vi "Transcriptor LabVIEW to Python code Step 3 Translate Elements.vi"(8 "error in (no error)":errorcluster, 10 "reentrant VIs":string[](array[string]), 11 "Diagram in":refnum<vi>) -> (0 "error out":errorcluster, 1 "transcripted C code":string[](array[string]), 2 "feedback assignments":string[](array[string]), 3 "transcriptor cluster":T1[](array[typedef]))   [LabVIEW 2018]
uses:
  types/LabVIEW Universal Transcriptor Cluster.ctl
  <vilib>/Utility/miscctls.llb/LVPointTypeDef.ctl
  <vilib>/regexp/Match Regular Expression.xnode
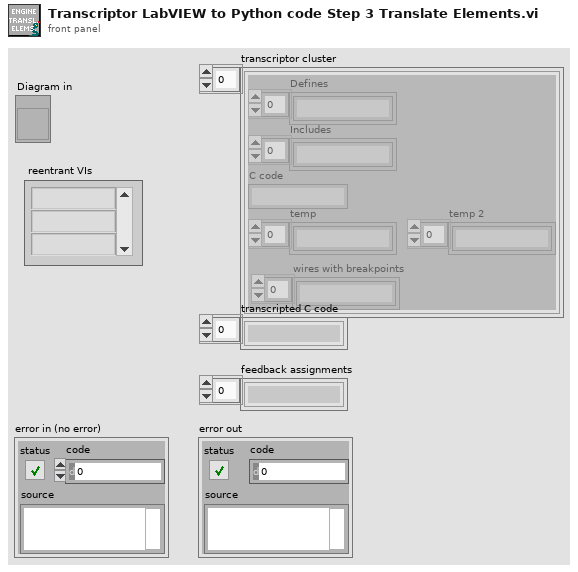
[diagram p1: front panel]
types:
  T1 = typedef "LabVIEW Universal Transcriptor Cluster.ctl" = cluster{"Defines":string[], "Includes":string[], "C code":string, "temp":string[], "temp 2":string[], "wires with breakpoints":string[]}
  T2 = typedef "LVPointTypeDef.ctl" = cluster{"Horizontal":i16, "Vertical":i16}
  T3 = cluster{"wire labels":string[], "wire terminals datatypes":string[][]}
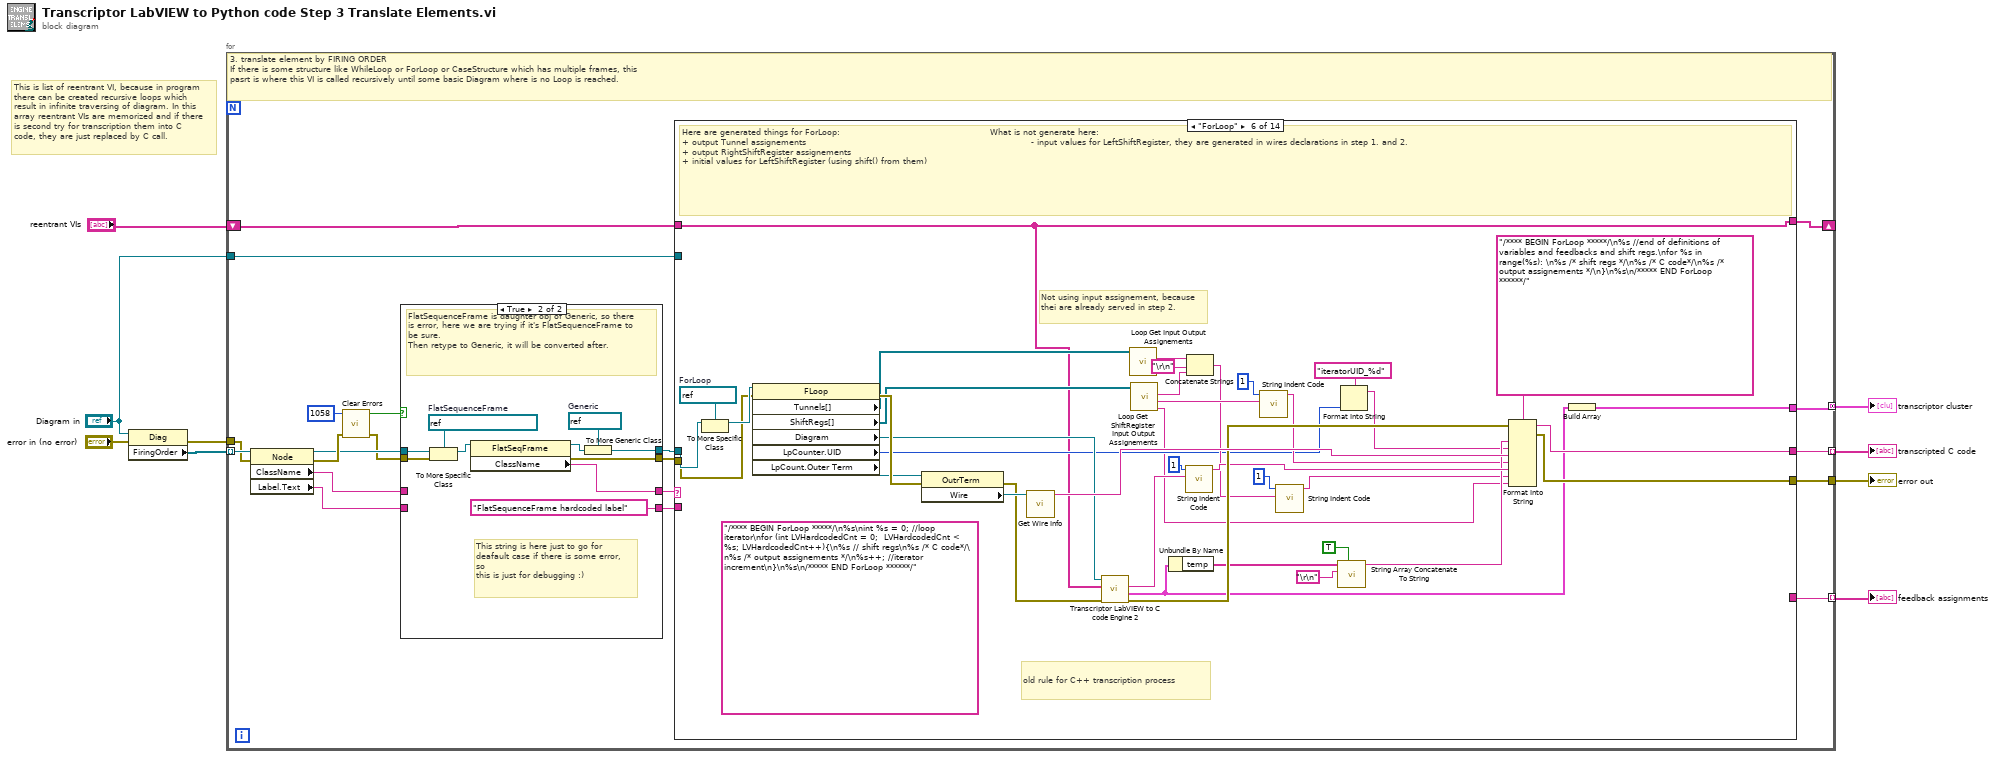
[diagram p0: block diagram]
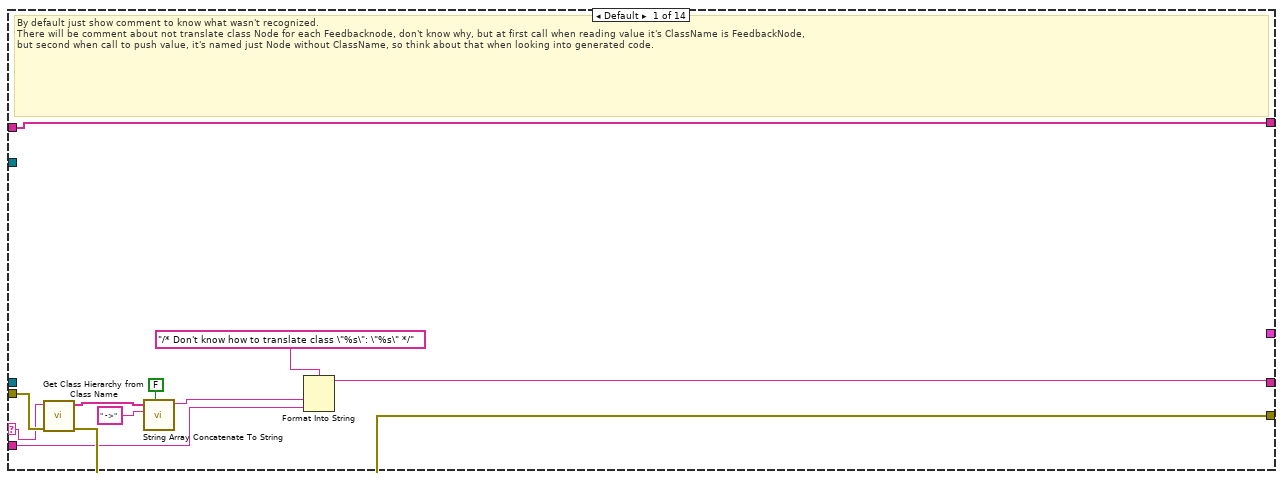
[diagram p3: hidden frame]
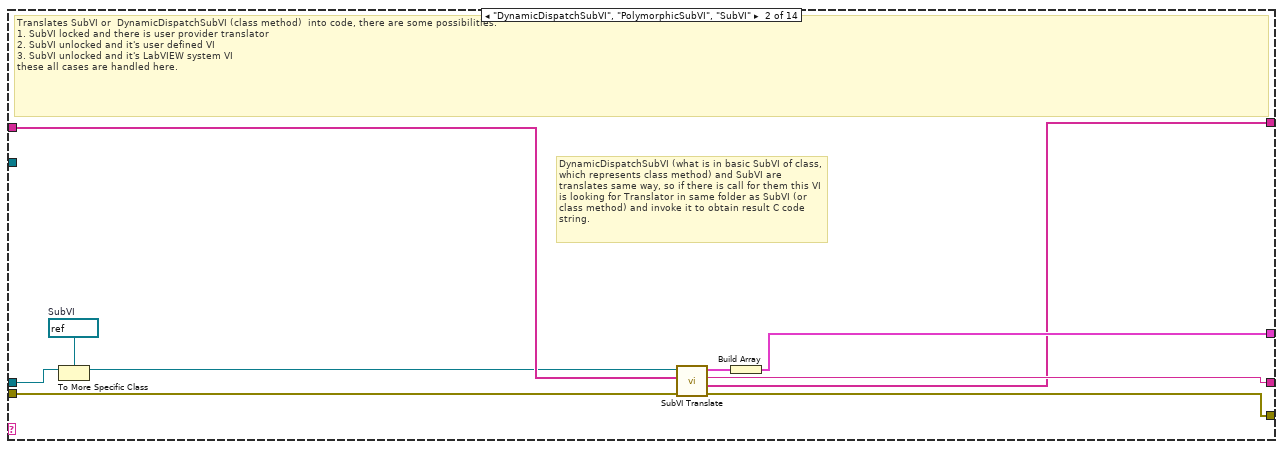
[diagram p4: hidden frame]
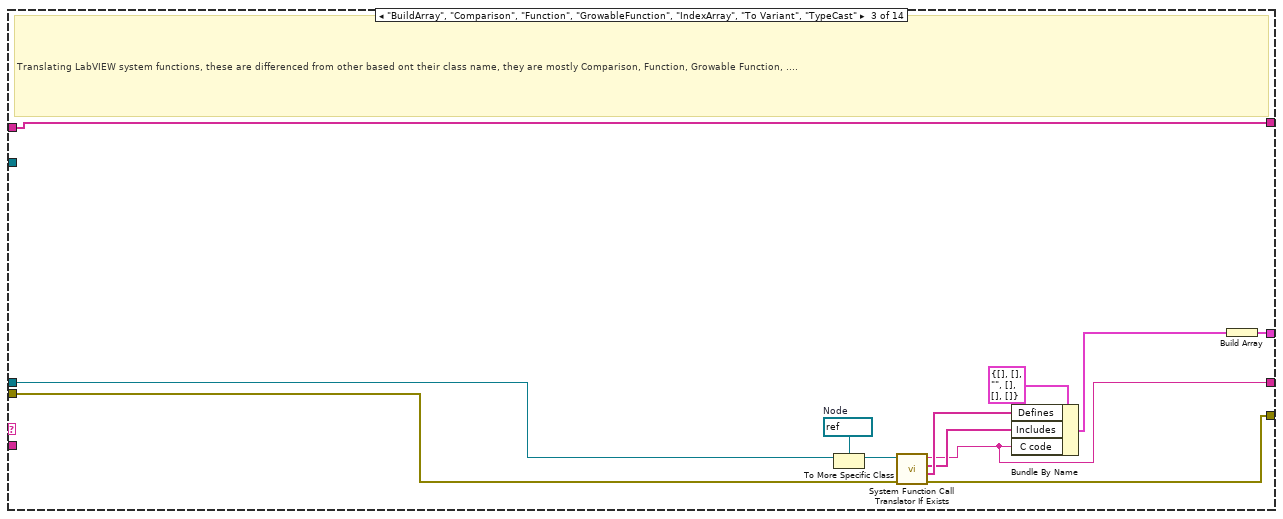
[diagram p5: hidden frame]
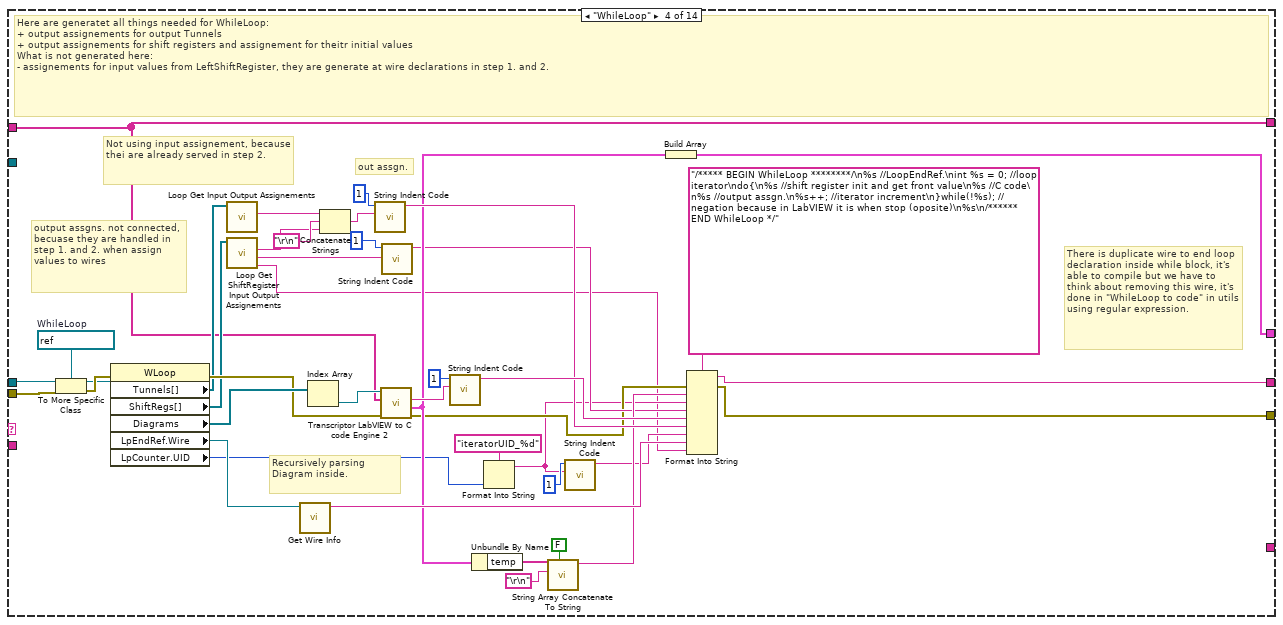
[diagram p6: hidden frame]
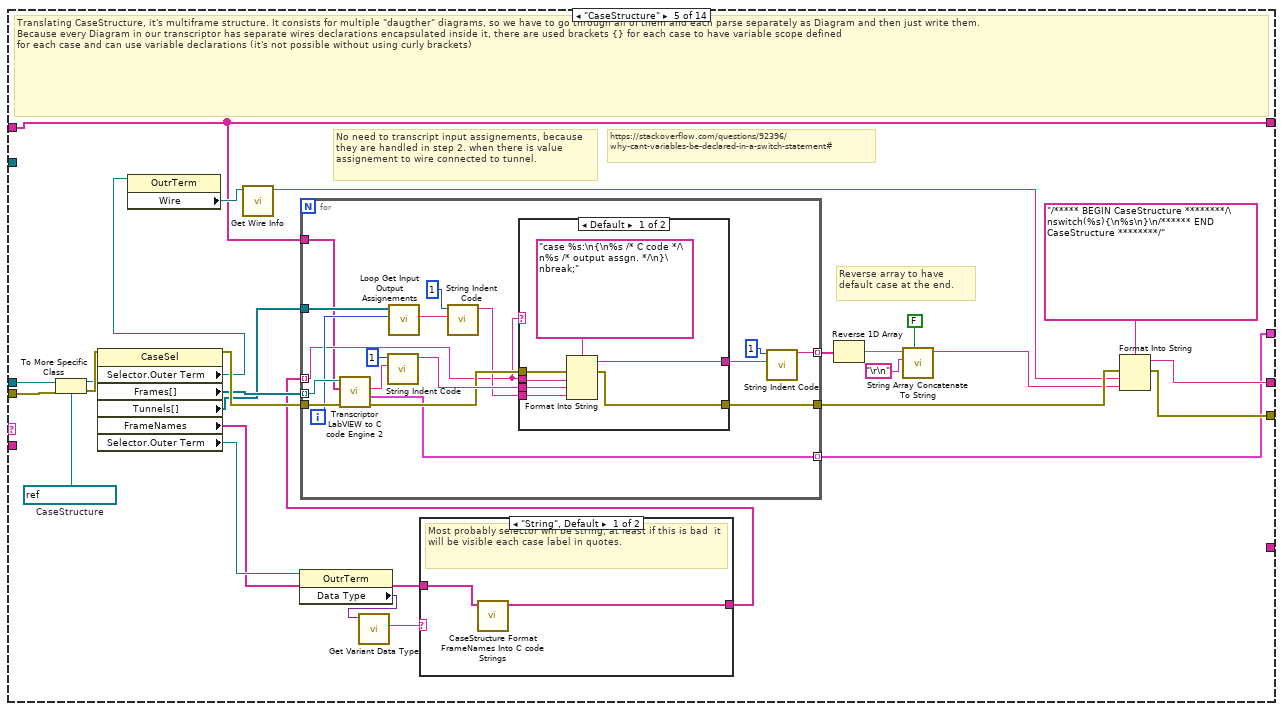
[diagram p7: hidden frame]
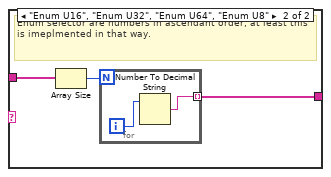
[diagram p8: hidden frame]
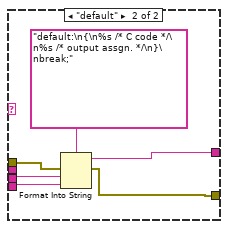
[diagram p9: hidden frame]
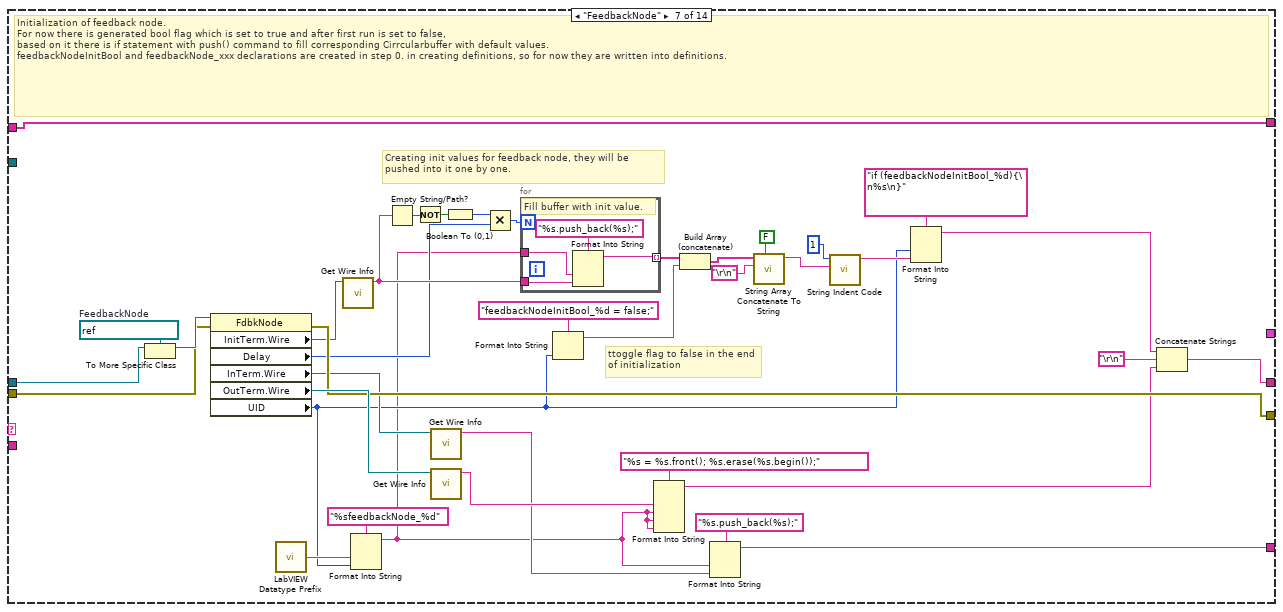
[diagram p10: hidden frame]
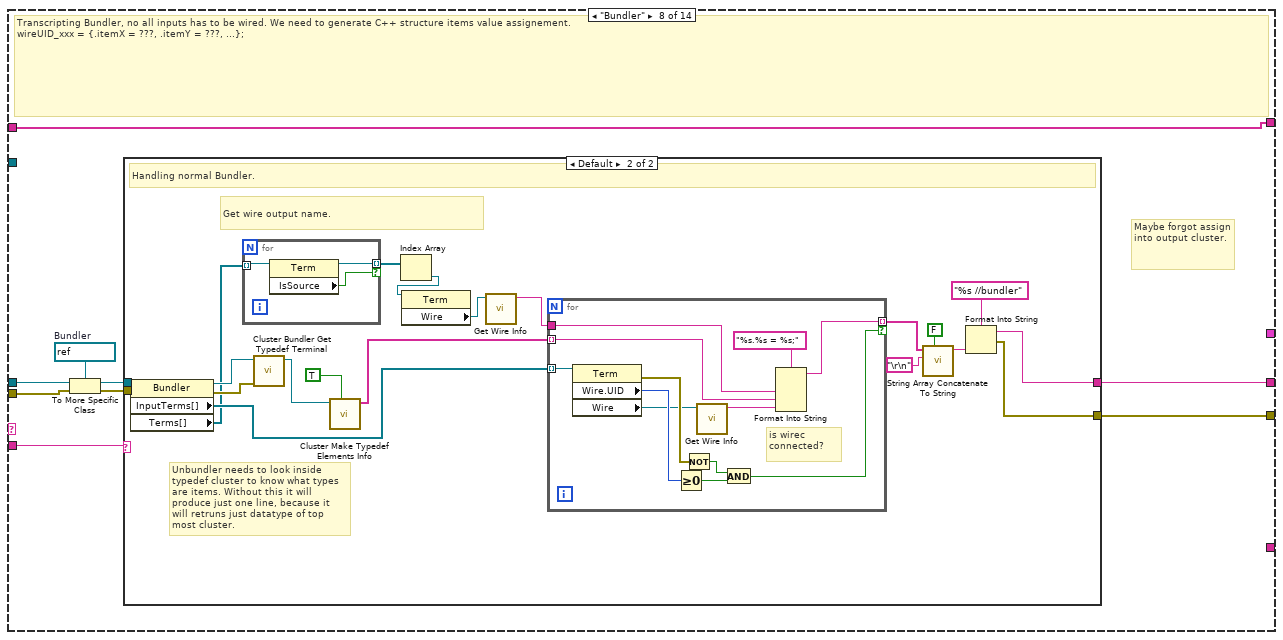
[diagram p11: hidden frame]
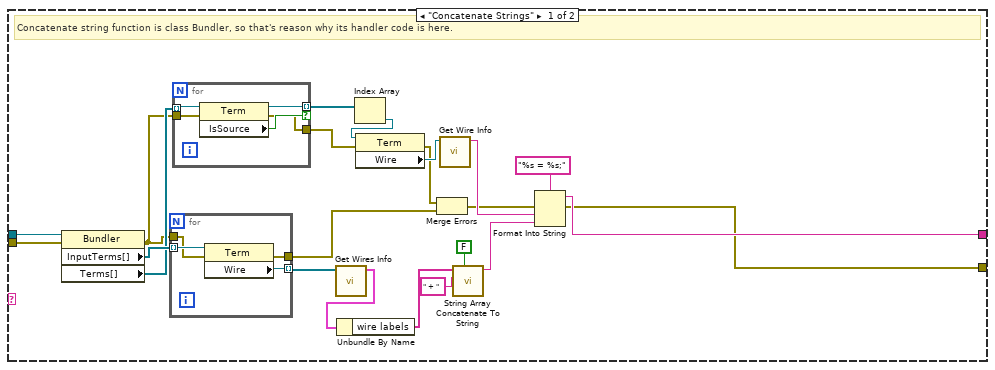
[diagram p12: hidden frame]
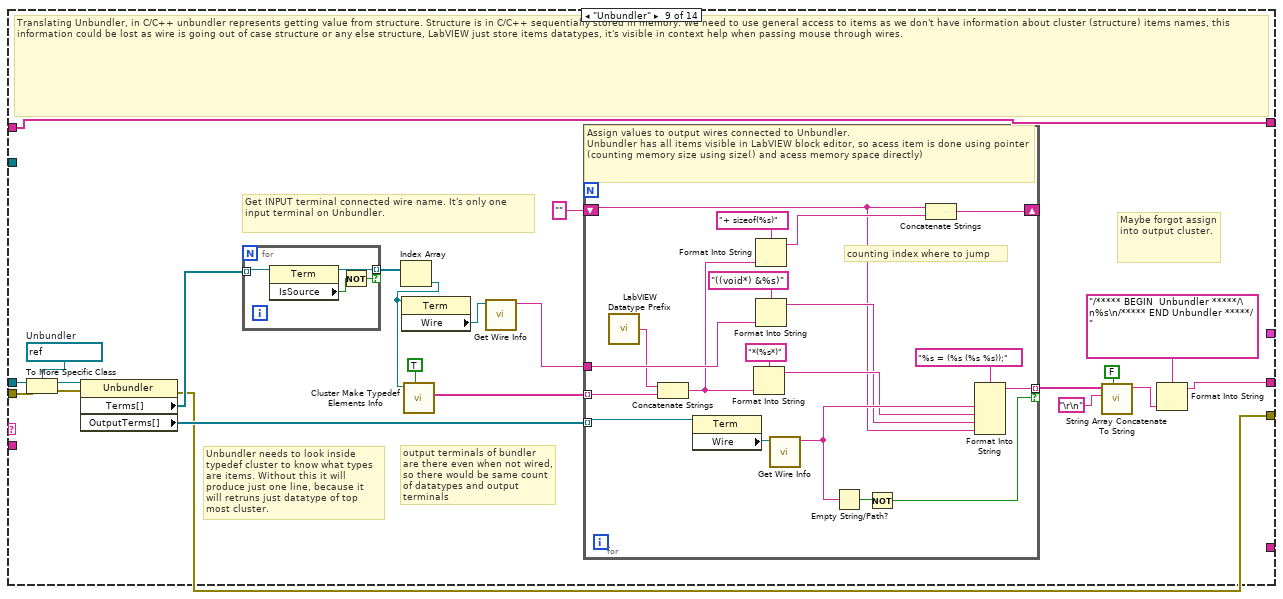
[diagram p13: hidden frame]
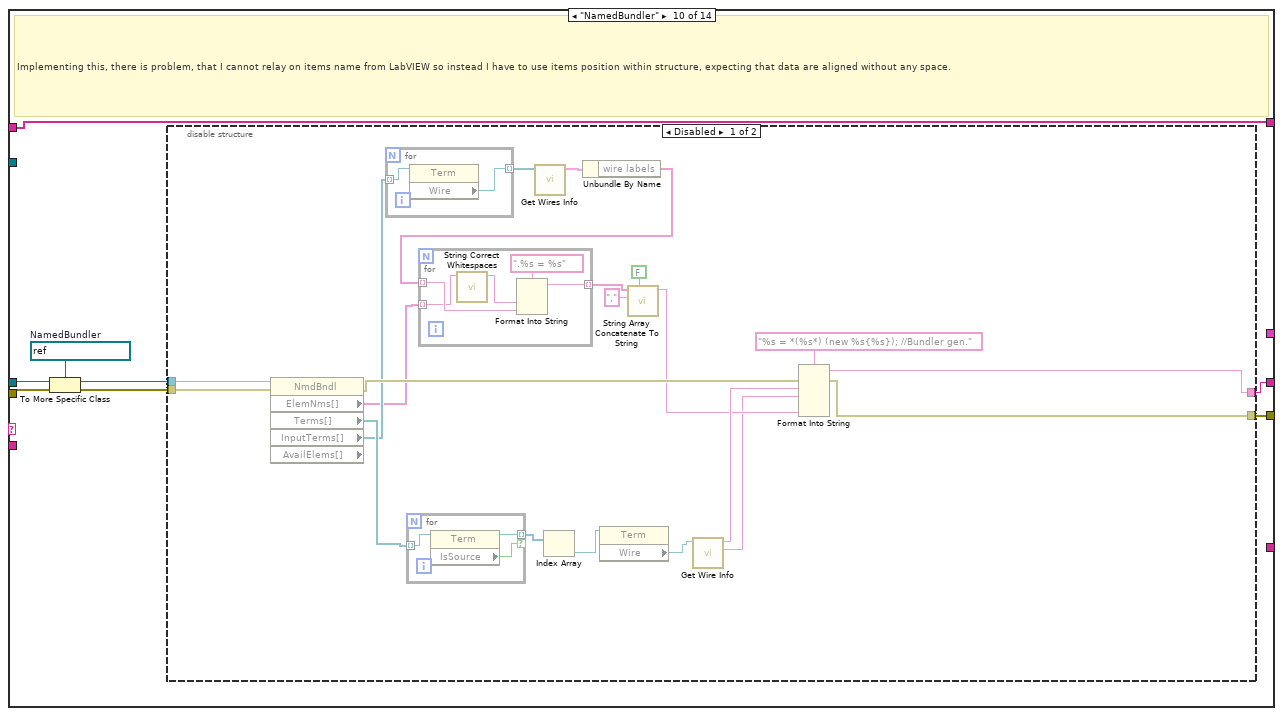
[diagram p14: hidden frame]
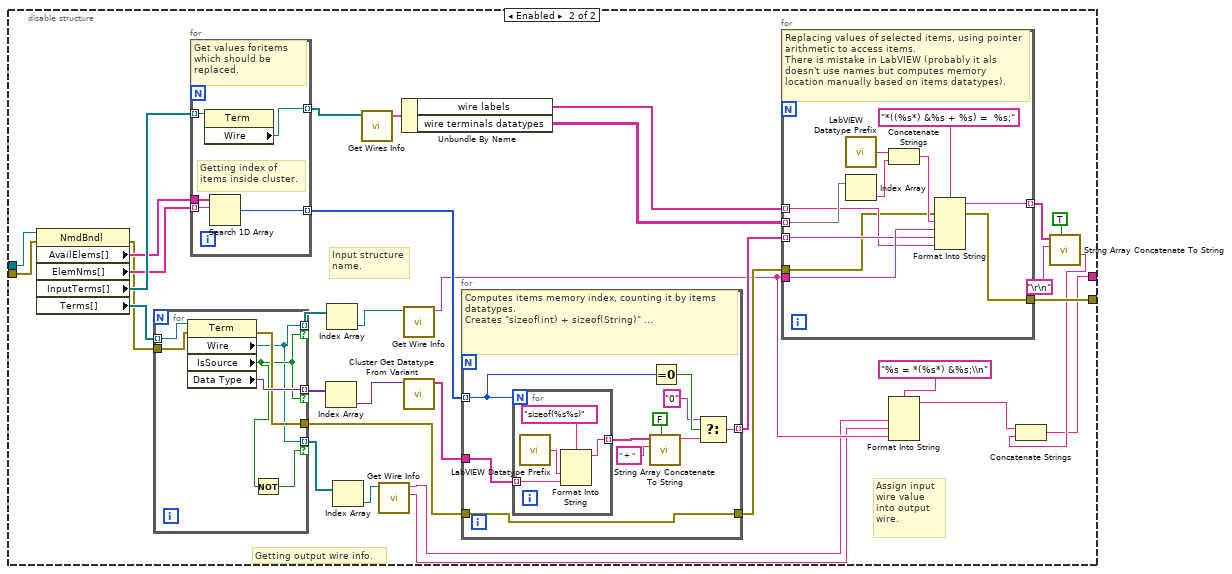
[diagram p15: hidden frame]
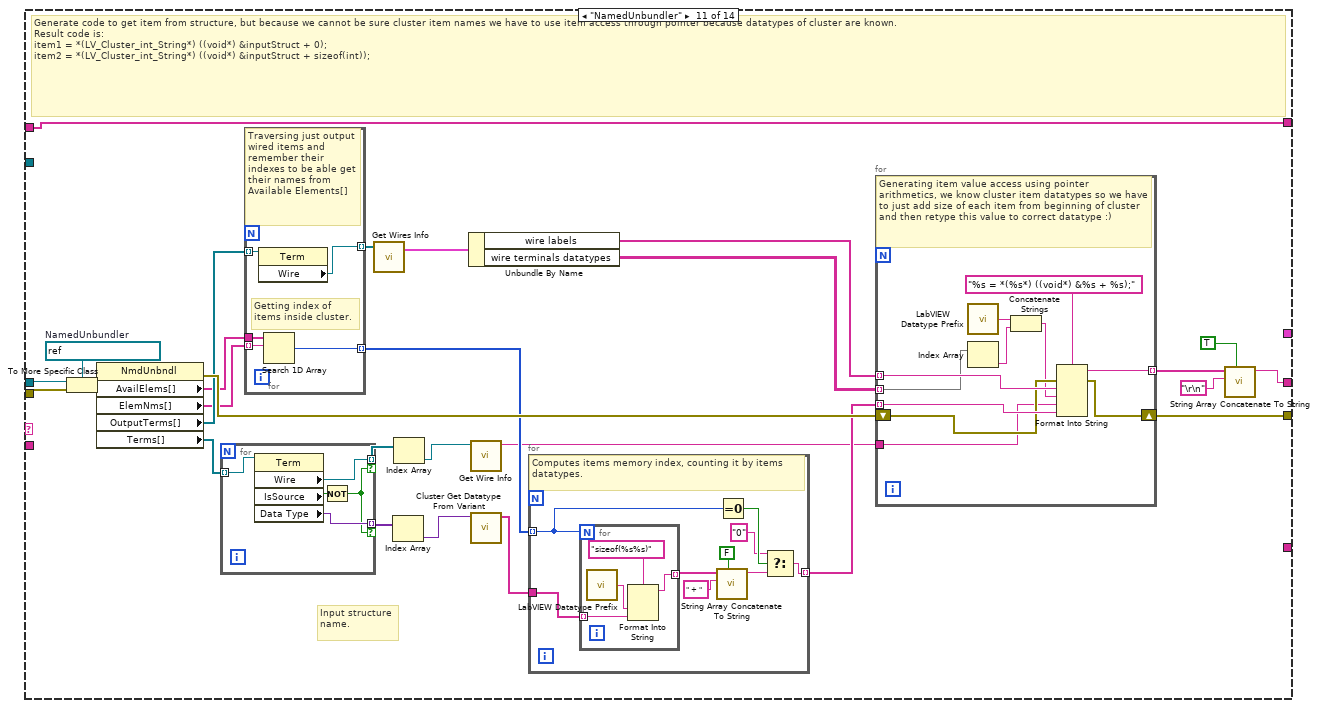
[diagram p16: hidden frame]
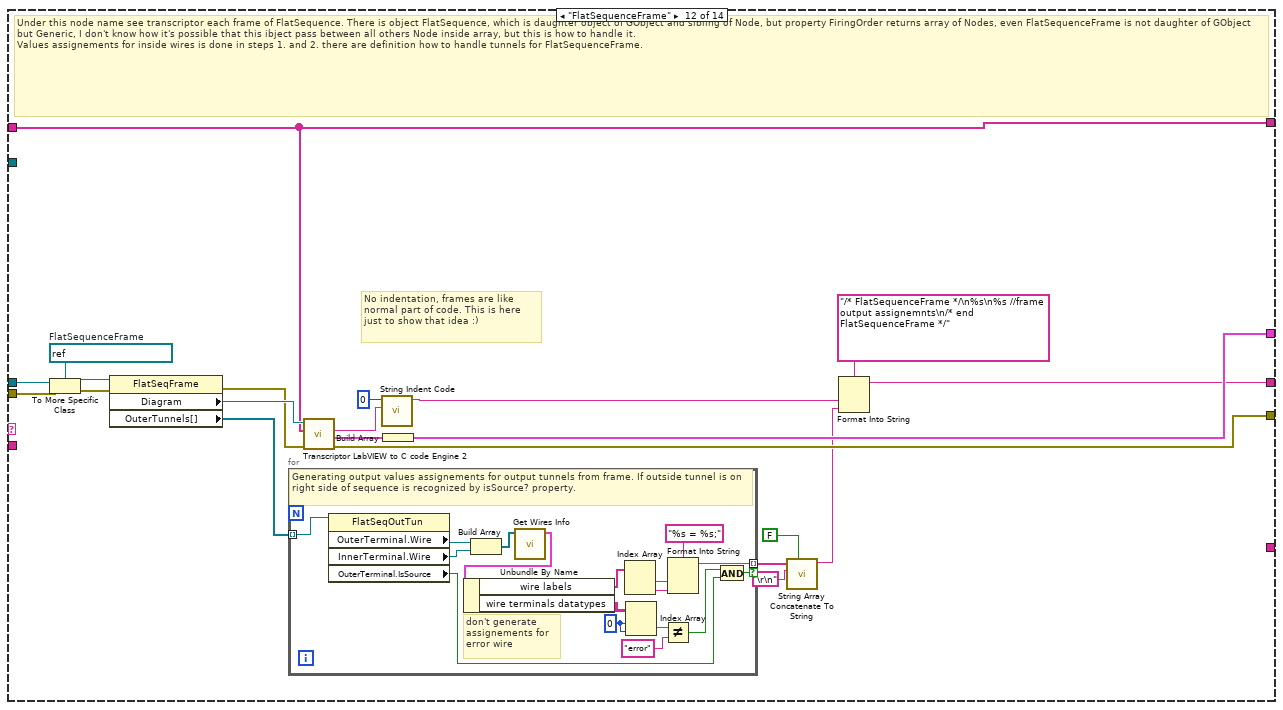
[diagram p17: hidden frame]
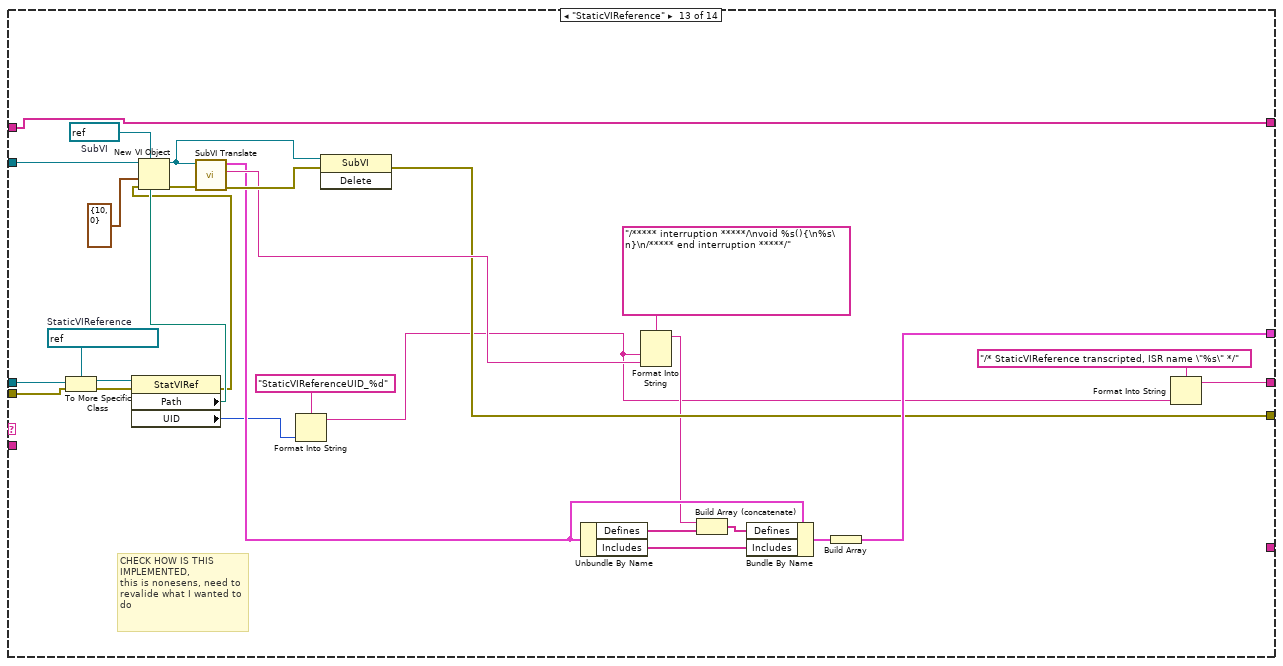
[diagram p18: hidden frame]
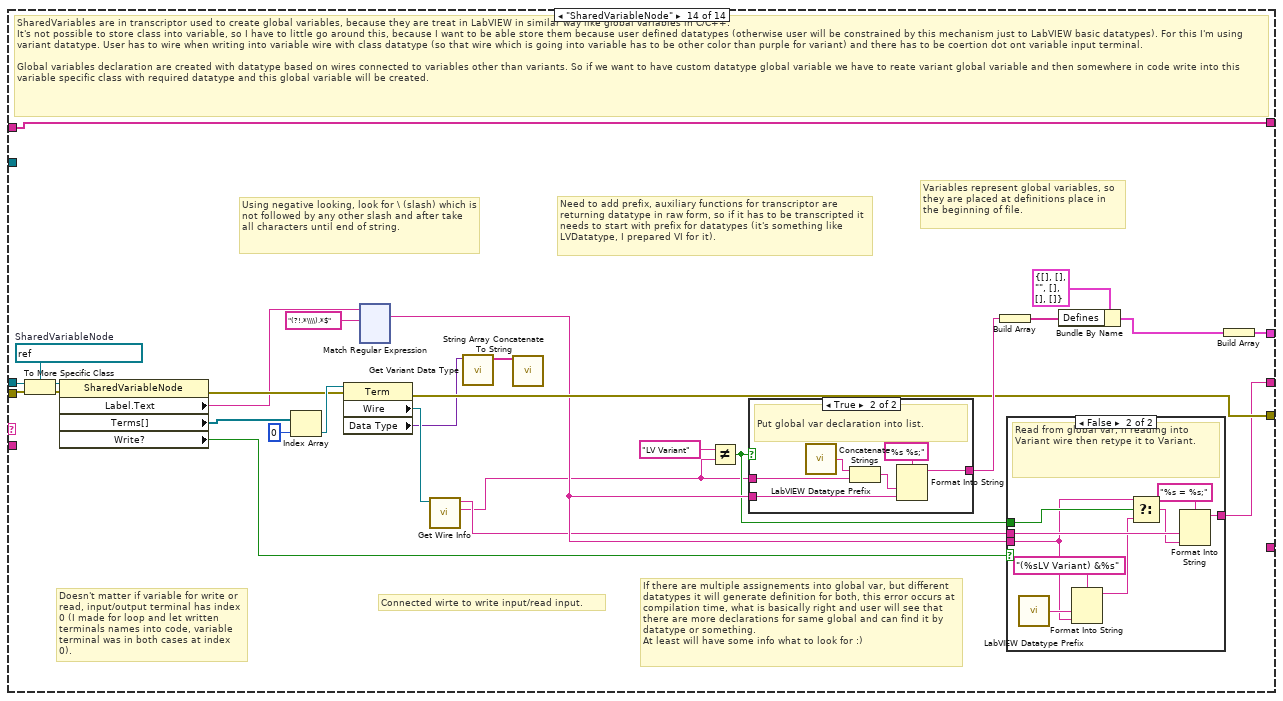
[diagram p19: hidden frame]
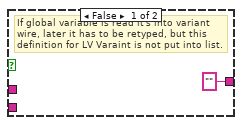
[diagram p20: hidden frame]
diagram:
  # "This is list of reentrant VI, because in program there can be created recursive loops which result in infinite traversing of diagram. In this array reentrant VIs are memorized and if there is second try for transcription them into C code, they are just replaced by C call."
  n1 = property on="Property Node" class="Diag"(reference="Diagram in", error in="error in (no error)") -> (error out=w4:errorcluster, "FiringOrder"=w9:refnum<vi>[])  [unwired: 1 out]
  n2 = for {
    tunnel: w9 -> [w29] mode=indexing
    tunnel: w4 -> [w28]
    tunnel: [w25] -> w5 mode=indexing
    tunnel: [w24] -> w7
    tunnel: [w27] -> w3 mode=concatenating
    tunnel: [w26] -> w8 mode=indexing
    tunnel: "Diagram in" -> [w12]
    shift-right: [w11] -> _
    shift-left: "reentrant VIs" -> [w10]
    # "3. translate element by FIRING ORDER\nIf there is some structure like WhileLoop or ForLoop or CaseStructure which has multiple frames, this\npasrt is where this VI is called recursively until some basic Diagram where is no Loop is reached."
    n3 = property class="Node"(reference=w29, error in=w28) -> (reference out=w21:refnum<vi>, error out=w23:errorcluster, "ClassName"=w16:string, "Label.Text"=w15:string)
    n4 = call <vilib>:"Clear Errors.vi"("error in (no error)"=w23, "specific error code to clear (0: all)"=1058) -> ("error out"=w20:errorcluster, "specific error cleared?"=w19:bool)  [unwired: 4 in]
    n5 = case shown="True" w19 {
      tunnel: w21 -> [w30 w43]
      tunnel: w20 -> [w31 w42]
      tunnel: [w33 w39] -> w18
      tunnel: [w32 "FlatSequenceFrame hardcoded label" ("Label.Text")] -> w17
      tunnel: w16 -> [w33 _]
      tunnel: w15 -> [w32 _]
      tunnel: [w31 w38] -> w14
      tunnel: [w30 w34] -> w13
      frame False {
        # "No error, so we are parsing some Node."
      }
      frame True {
        w36 = refnum<vi> refnum  # Generic
        w41 = refnum<vi> refnum  # FlatSequenceFrame
        # "This string is here just to go for\ndeafault case if there is some error, so\nthis is just for debugging :)"
        # "FlatSequenceFrame is daughter obj of Generic, so there is error, here we are trying if it's FlatSequenceFrame to be sure.\nThen retype to Generic, it will be converted after."
        n6 = To More Specific Class(target class=w41, reference=w43, error in=w42) -> (specific class reference=w40:refnum<vi>)  [unwired: 1 out]
        n7 = property class="FlatSeqFrame"(reference=w40) -> (reference out=w35:refnum<vi>, error out=w38:errorcluster, "ClassName"=w39:string)  [unwired: 1 in]
        n8 = To More Generic Class(target class=w36, reference=w35) -> (generic class reference=w34:refnum<vi>)
      }
    }
    n9 = case shown="\"ForLoop\"" w18 {
      selector: w18 -> [w45 _ _ _ _ _ _ _ _ _ _ _ _ _]
      tunnel: w13 -> [_ w57 w68 w117 w127 w221 w259 w271 w357 w391 w520 w575 w620 w648]
      tunnel: [w53 w64 w73 w109 w139 w211 w232 w266 w341 w385 w506 w561 w597 w626] -> w25
      tunnel: w14 -> [w48 w60 w76 w113 w142 w218 w251 w270 w356 w390 w519 w571 w619 w649]
      tunnel: [w47 w63 w70 w108 w137 w212 w250 w267 w344 w386 w514 w565 w605 w636] -> w24
      tunnel: [_ w61 w72 w98 w126 w203 _ _ _ _ _ w563 w616 w642] -> w27
      tunnel: w17 -> [w46 _ _ _ _ _ _ w265 _ _ _ _ _ _]
      tunnel: [_ _ _ _ _ _ w226 _ _ _ _ _ _ _] -> w26
      tunnel: w12 -> [_ _ _ _ _ _ _ _ _ _ _ _ w614 _]
      tunnel: w10 -> [w44 w59 w65 w78 w123 w184 w222 w264 w340 w384 w493 w555 w593 w644]
      tunnel: [w44 w58 w65 w78 w123 w184 w222 w264 w340 w384 w493 w555 w593 w644] -> w11
      frame Default {
        # "By default just show comment to know what wasn't recognized.\nThere will be comment about not translate class Node for each Feedbacknode, don't know why, but at first call when reading value it's ClassName is FeedbackNode,\nbut second when call to push value, it's named just Node without ClassName, so think about that when looking into generated code."
        n10 = call <vilib>:"Get Class Hierarchy from Class Name.vi"("error in (no error)"=w48, "Class Name"=w45) -> ("error out"=w47:errorcluster, "Class Hierarchy"=w51:string[])  [unwired: 8 in]
        n11 = call "String Array Concatenate To String.vi"("insert last delimiter?"=FALSE, "Delimiter char"=" ->", "Array String In"=w51) -> ("String"=w49:string)  [unwired: 8 in]
        n12 = Format Into String(format string="/* Don't know how to translate class \"%s\": \"%s\" */", w49, w46) -> (resulting string=w53:string)  [unwired: 2 in, 1 out]
      }
      frame "DynamicDispatchSubVI", "PolymorphicSubVI", "SubVI" {
        w55 = refnum<vi> refnum  # SubVI
        # "DynamicDispatchSubVI (what is in basic SubVI of class, which represents class method) and SubVI are translates same way, so if there is call for them this VI is looking for Translator in same folder as SubVI (or class method) and invoke it to obtain result C code string."
        # "Translates SubVI or  DynamicDispatchSubVI (class method)  into code, there are some possibilities:\n1. SubVI locked and there is user provider translator\n2. SubVI unlocked and it's user defined VI\n3. SubVI unlocked and it's LabVIEW system VI\nthese all cases are handled here."
        n13 = To More Specific Class(target class=w55, reference=w57) -> (specific class reference=w56:refnum<vi>)  [unwired: 1 in, 1 out]
        n14 = call "SubVI Translate.vi"("error in (no error)"=w60, "reentrant VIs"=w59, "SubVI in"=w56) -> ("error out"=w63:errorcluster, "reentrant VIs out"=w58:string[], "transcripted code"=w64:string, "transcriptor cluster"=w62:T1)  [unwired: 5 in]
        n15 = Build Array(w62) -> (w61:T1[])
      }
      frame "BuildArray", "Comparison", "Function", "GrowableFunction", "IndexArray", "To Variant", "TypeCast" {
        w66 = refnum<vi> refnum  # Node
        # "Translating LabVIEW system functions, these are differenced from other based ont their class name, they are mostly Comparison, Function, Growable Function, ...."
        n16 = To More Specific Class(target class=w66, reference=w68) -> (specific class reference=w67:refnum<vi>)  [unwired: 1 in, 1 out]
        n17 = call "System Function Call Translator If Exists.vi"("Error In"=w76, "Node Refnum"=w67) -> ("Error Out"=w70:errorcluster, "Defines"=w75:string[], "Includes"=w74:string[], "Replaced Code"=w73:string)  [unwired: 6 in]
        n18 = Bundle By Name(cluster=T1 {"Defines"=[], "Includes"=[], "C code"="", "temp"=[], "temp 2"=[], "wires with breakpoints"=[]} ("input cluster"), "Defines"=w75, "Includes"=w74, "C code"=w73) -> (w71:T1)
        n19 = Build Array(w71) -> (w72:T1[])
      }
      frame "WhileLoop" {
        w116 = refnum<vi> refnum  # WhileLoop
        # "output assgns. not connected, becuase they are handled in step 1. and 2. when assign values to wires"
        # "Not using input assignement, because thei are already served in step 2."
        # "out assgn."
        # "There is duplicate wire to end loop declaration inside while block, it's able to compile but we have to think about removing this wire, it's done in \"WhileLoop to code\" in utils using regular expression."
        # "Recursively parsing Diagram inside."
        # "Here are generatet all things needed for WhileLoop:\n+ output assignements for output Tunnels\n+ output assignements for shift registers and assignement for theitr initial values\nWhat is not generated here:\n- assignements for input values from LeftShiftRegister, they are generate at wire declarations in step 1. and 2."
        n20 = To More Specific Class(target class=w116, reference=w117, error in=w113) -> (specific class reference=w107:refnum<vi>, error out=w115:errorcluster)
        n21 = property class="WLoop"(reference=w107, error in=w115) -> (error out=w112:errorcluster, "Tunnels[]"=w102:refnum<vi>[], "ShiftRegs[]"=w89:refnum<vi>[], "Diagrams"=w114:refnum<vi>[], "LpEndRef.Wire"=w106:refnum<vi>, "LpCounter.UID"=w82:i32)  [unwired: 1 out]
        n22 = call "Loop Get Input Output Assignements.vi"("Loop Tunnels[]"=w102) -> ("tunnels output assignements"=w93:string)  [unwired: 9 in, 1 out]
        n23 = call "Loop Get ShiftRegister Input Output Assignements.vi"("RightShiftRegister[]"=w89) -> ("right shift regs outside wires assgn."=w77:string, "init values"=w79:string, "output assignements"=w88:string)  [unwired: 7 in, 1 out]
        n24 = call "Get Wire Info.vi"("Wire"=w106) -> ("wire label"=w101:string)  [unwired: 9 in, 1 out]
        n25 = Index Array(array=w114) -> (element=w111:refnum<vi>)  [unwired: 1 in]
        n26 = Concatenate Strings(w93, "\r\n", w88) -> (w91:string)
        n27 = call "String Indent Code.vi"("complete code"=w91, "actual nested level"=1) -> ("indented code"=w99:string)  [unwired: 9 in]
        n28 = call "Transcriptor LabVIEW to C code Engine 2.vi"("Error In"=w112, "List Reentrant VIs"=w78, "Diagram in"=w111) -> ("error out"=w85:errorcluster, "output cluster"=w97:T1, "transcripted code"=w105:string)  [unwired: 4 in, 2 out]
        n29 = call "String Indent Code.vi"("complete code"=w79, "actual nested level"=1) -> ("indented code"=w86:string)  [unwired: 9 in]
        n30 = call "String Indent Code.vi"("complete code"=w105, "actual nested level"=1) -> ("indented code"=w103:string)  [unwired: 9 in]
        n31 = Unbundle By Name(w97) -> ("temp"=w96:string[])
        n32 = Format Into String(format string="iteratorUID_%d", w82) -> (resulting string=w80:string)  [unwired: 2 in, 1 out]
        n33 = call "String Array Concatenate To String.vi"("insert last delimiter?"=FALSE, "Delimiter char"="\r\n", "Array String In"=w96) -> ("String"=w90:string)  [unwired: 8 in]
        n34 = call "String Indent Code.vi"("complete code"=w80, "actual nested level"=1) -> ("indented code"=w81:string)  [unwired: 9 in]
        n35 = Build Array(w97) -> (w98:T1[])
        n36 = Format Into String(format string="/***** BEGIN WhileLoop ********/\n%s //LoopEndRef.\nint %s = 0; //loop iterator\ndo{\n%s //shift register init and get front value\n%s //C code\n%s //output assgn.\n%s++; //iterator increment\n}while(!%s); //negation because in LabVIEW it is when stop (oposite)\n%s\n/****** END WhileLoop */", error in=w85, w90, w80, w86, w103, w99, w81, w101, w77) -> (resulting string=w109:string, error out=w108:errorcluster)  [unwired: 1 in]
      }
      frame "CaseStructure" {
        w144 = refnum<vi> refnum  # CaseStructure
        # "Reverse array to have default case at the end."
        # "https://stackoverflow.com/questions/92396/why-cant-variables-be-declared-in-a-switch-statement#"
        # "No need to transcript input assignements, because they are handled in step 2. when there is value assignement to wire connected to tunnel."
        # "Translating CaseStructure, it's multiframe structure. It consists for multiple \"daugther\" diagrams, so we have to go through all of them and each parse separately as Diagram and then just write them.\nBecause every Diagram in our transcriptor has separate wires declarations encapsulated inside it, there are used brackets {} for each case to have variable scope defined\nfor each case and can use variable declarations (it's not possible without using curly brackets)"
        n37 = To More Specific Class(target class=w144, reference=w127, error in=w142) -> (specific class reference=w136:refnum<vi>, error out=w143:errorcluster)
        n38 = property class="CaseSel"(reference=w136, error in=w143) -> (error out=w141:errorcluster, "Selector.Outer Term"=w134:refnum<vi>, "Frames[]"=w135:refnum<vi>[], "Tunnels[]"=w128:refnum<vi>[], "FrameNames"=w119:string[], "Selector.Outer Term"=w122:refnum<vi>)  [unwired: 1 out]
        n39 = property class="OutrTerm"(reference=w134) -> ("Wire"=w133:refnum<vi>)  [unwired: 1 in, 2 out]
        n40 = call "Get Wire Info.vi"("Wire"=w133) -> ("wire label"=w132:string)  [unwired: 9 in, 1 out]
        n41 = property class="OutrTerm"(reference=w122) -> ("Data Type"=w121:variant)  [unwired: 1 in, 2 out]
        n42 = call "Get Variant Data Type.vi"("Variant in"=w121) -> ("first data type"=w120:string)  [unwired: 9 in, 1 out]
        n43 = case shown="\"String\", Default" w120 {
          tunnel: w119 -> [w146 w149]
          tunnel: [w145 w147] -> w118
          frame "String", Default {
            # "Most probably selector will be string, at least if this is bad  it will be visible each case label in quotes."
            n44 = call "CaseStructure Format FrameNames Into C code Strings.vi"("FrameNames in"=w146) -> ("c code cases names"=w145:string[])  [unwired: 10 in]
          }
          frame "Enum U16", "Enum U32", "Enum U64", "Enum U8" {
            # "Enum selector are numbers in ascendant order, at least this is imeplmented in that way."
            n45 = Array Size(array=w149) -> (size(s)=w148:i32)
            n46 = for {
              N: w148 -> [_]
              tunnel: [w150] -> w147 mode=indexing
              i -> [w151]
              n47 = Number To Decimal String(number=w151) -> (decimal integer string=w150:string)  [unwired: 1 in]
            }
          }
        }
        n48 = for {
          tunnel: w141 -> [w169]
          tunnel: [w163] -> w138
          tunnel: w135 -> [w168] mode=indexing
          tunnel: w118 -> [w153] mode=indexing
          tunnel: [w161] -> w125 mode=indexing
          tunnel: w128 -> [w158]
          tunnel: [w154] -> w126 mode=indexing
          tunnel: w123 -> [w152]
          i -> [w159]
          n49 = call "Transcriptor LabVIEW to C code Engine 2.vi"("Error In"=w169, "List Reentrant VIs"=w152, "Diagram in"=w168) -> ("error out"=w164:errorcluster, "output cluster"=w154:T1, "transcripted code"=w166:string)  [unwired: 4 in, 2 out]
          n50 = call "String Indent Code.vi"("complete code"=w166, "actual nested level"=1) -> ("indented code"=w165:string)  [unwired: 9 in]
          n51 = call "Loop Get Input Output Assignements.vi"("Inside Terms[] offset"=w159, "Loop Tunnels[]"=w158) -> ("tunnels output assignements"=w156:string)  [unwired: 8 in, 1 out]
          n52 = call "String Indent Code.vi"("complete code"=w156, "actual nested level"=1) -> ("indented code"=w155:string)  [unwired: 9 in]
          n53 = case shown="Default" w153 {
            tunnel: w165 -> [w176 w178]
            tunnel: w153 -> [w175 _]
            tunnel: w164 -> [w173 w177]
            tunnel: [w172 w180] -> w163
            tunnel: [w171 w181] -> w160
            tunnel: w155 -> [w170 w179]
            frame Default {
              n54 = Format Into String(format string="case %s:\n{\n%s /* C code */\n%s /* output assgn. */\n}\nbreak;", error in=w173, w175, w176, w170) -> (resulting string=w171:string, error out=w172:errorcluster)  [unwired: 1 in]
            }
            frame "default" {
              n55 = Format Into String(format string="default:\n{\n%s /* C code */\n%s /* output assgn. */\n}\nbreak;", error in=w177, w178, w179) -> (resulting string=w181:string, error out=w180:errorcluster)  [unwired: 1 in]
            }
          }
          n56 = call "String Indent Code.vi"("complete code"=w160, "actual nested level"=1) -> ("indented code"=w161:string)  [unwired: 9 in]
        }
        n57 = Reverse 1D Array(array=w125) -> (reversed array=w124:string[])
        n58 = call "String Array Concatenate To String.vi"("insert last delimiter?"=FALSE, "Delimiter char"="\r\n", "Array String In"=w124) -> ("String"=w129:string)  [unwired: 8 in]
        n59 = Format Into String(format string="/***** BEGIN CaseStructure ********/\nswitch(%s){\n%s\n}\n/****** END CaseStructure ********/", error in=w138, w132, w129) -> (resulting string=w139:string, error out=w137:errorcluster)  [unwired: 1 in]
      }
      frame "ForLoop" {
        (unwired) "/**** BEGIN ForLoop *****/\n%s\nint %s = 0; //loop iterator\nfor (int LVHardcodedCnt = 0;  LVHardcodedCnt < %s; LVHardcodedCnt++){\n%s // shift regs\n%s /* C code*/\n%s /* output assignements */\n%s++; //iterator increment\n}\n%s\n/***** END ForLoop ******/" ("format string")
        w220 = refnum<vi> refnum  # ForLoop
        # "old rule for C++ transcription process"
        # "Not using input assignement, because thei are already served in step 2."
        # "Here are generated things for ForLoop:                                                  What is not generate here:\n+ output Tunnel assignements                                                                           - input values for LeftShiftRegister, they are generated in wires declarations in step 1. and 2.\n+ output RightShiftRegister assignements\n+ initial values for LeftShiftRegister (using shift() from them)"
        n60 = To More Specific Class(target class=w220, reference=w221) -> (specific class reference=w219:refnum<vi>)  [unwired: 1 in, 1 out]
        n61 = property class="FLoop"(reference=w219, error in=w218) -> (error out=w217:errorcluster, "Tunnels[]"=w204:refnum<vi>[], "ShiftRegs[]"=w197:refnum<vi>[], "Diagram"=w210:refnum<vi>, "LpCounter.UID"=w186:i32, "LpCount.Outer Term"=w216:refnum<vi>)  [unwired: 1 out]
        n62 = property class="OutrTerm"(reference=w216, error in=w217) -> (error out=w209:errorcluster, "Wire"=w215:refnum<vi>)  [unwired: 1 out]
        n63 = call "Get Wire Info.vi"("Wire"=w215) -> ("wire label"=w213:string)  [unwired: 9 in, 1 out]
        n64 = call "Transcriptor LabVIEW to C code Engine 2.vi"("Error In"=w209, "List Reentrant VIs"=w184, "Diagram in"=w210) -> ("error out"=w208:errorcluster, "output cluster"=w202:T1, "transcripted code"=w207:string)  [unwired: 4 in, 2 out]
        n65 = call "Loop Get Input Output Assignements.vi"("Loop Tunnels[]"=w204) -> ("tunnels output assignements"=w194:string)  [unwired: 9 in, 1 out]
        n66 = call "Loop Get ShiftRegister Input Output Assignements.vi"("RightShiftRegister[]"=w197) -> ("right shift regs outside wires assgn."=w183:string, "init values"=w193:string, "output assignements"=w191:string)  [unwired: 7 in, 1 out]
        n67 = Unbundle By Name(w202) -> ("temp"=w201:string[])
        n68 = call "String Indent Code.vi"("complete code"=w207, "actual nested level"=1) -> ("indented code"=w205:string)  [unwired: 9 in]
        n69 = Concatenate Strings(w194, "\r\n", w191) -> (w189:string)
        n70 = call "String Indent Code.vi"("complete code"=w193, "actual nested level"=1) -> ("indented code"=w195:string)  [unwired: 9 in]
        n71 = call "String Indent Code.vi"("complete code"=w189, "actual nested level"=1) -> ("indented code"=w188:string)  [unwired: 9 in]
        n72 = call "String Array Concatenate To String.vi"("insert last delimiter?"=TRUE, "Delimiter char"="\r\n", "Array String In"=w201) -> ("String"=w198:string)  [unwired: 8 in]
        n73 = Format Into String(format string="iteratorUID_%d", w186) -> (resulting string=w185:string)  [unwired: 2 in, 1 out]
        n74 = Format Into String(format string="/**** BEGIN ForLoop *****/\n%s //end of definitions of variables and feedbacks and shift regs.\nfor %s in range(%s): \n%s /* shift regs */\n%s /* C code*/\n%s /* output assignements */\n}\n%s\n/***** END ForLoop ******/", error in=w208, w198, w185, w213, w195, w205, w188, w183) -> (resulting string=w211:string, error out=w212:errorcluster)  [unwired: 1 in]
        n75 = Build Array(w202) -> (w203:T1[])
      }
      frame "FeedbackNode" {
        w257 = refnum<vi> refnum  # FeedbackNode
        # "Creating init values for feedback node, they will be pushed into it one by one."
        # "ttoggle flag to false in the end of initialization"
        # "Initialization of feedback node.\nFor now there is generated bool flag which is set to true and after first run is set to false,\nbased on it there is if statement with push() command to fill corresponding Cirrcularbuffer with default values.\nfeedbackNodeInitBool and feedbackNode_xxx declarations are created in step 0. in creating definitions, so for now they are written into definitions."
        n76 = To More Specific Class(target class=w257, reference=w259) -> (specific class reference=w258:refnum<vi>)  [unwired: 1 in, 1 out]
        n77 = property class="FdbkNode"(reference=w258, error in=w251) -> (error out=w250:errorcluster, "InitTerm.Wire"=w244:refnum<vi>, "Delay"=w225:i32, "InTerm.Wire"=w245:refnum<vi>, "OutTerm.Wire"=w256:refnum<vi>, "UID"=w236:i32)  [unwired: 1 out]
        n78 = call "LabVIEW Datatype Prefix.vi"() -> ("datatype prefix"=w253:string)
        n79 = call "Get Wire Info.vi"("Wire"=w244) -> ("wire label"=w246:string)  [unwired: 9 in, 1 out]
        n80 = Format Into String(format string="%sfeedbackNode_%d" ("Replaced Code"), w253, w236) -> (resulting string=w223:string)  [unwired: 2 in, 1 out]
        n81 = Empty String/Path?(string/path=w246) -> (empty?=w249:bool)
        n82 = Not(x=w249) -> (.not. x?=w248:bool)
        n83 = call "Get Wire Info.vi"("Wire"=w245) -> ("wire label"=w227:string)  [unwired: 9 in, 1 out]
        n84 = call "Get Wire Info.vi"("Wire"=w256) -> ("wire label"=w252:string)  [unwired: 9 in, 1 out]
        n85 = Boolean To (0,1)(Boolean=w248) -> (0, 1=w224:i16)
        n86 = Multiply(x=w224, y=w225) -> (x*y=w247:i32)
        n87 = for {
          N: w247 -> [_]
          tunnel: [w262] -> w235 mode=indexing
          tunnel: w223 -> [w261]
          tunnel: w246 -> [w260]
          # "Fill buffer with init value."
          n88 = Format Into String(format string="%s.push_back(%s);", w261, w260) -> (resulting string=w262:string)  [unwired: 2 in, 1 out]
        }
        n89 = Format Into String(format string="feedbackNodeInitBool_%d = false;", w236) -> (resulting string=w234:string)  [unwired: 2 in, 1 out]
        n90 = Format Into String(format string="%s = %s.front(); %s.erase(%s.begin());" ("Replaced Code"), w252, w223, w223, w223) -> (resulting string=w230:string)  [unwired: 2 in, 1 out]
        n91 = Build Array (concatenate)(w235, w234) -> (w233:string[])
        n92 = Format Into String(format string="%s.push_back(%s);" ("Replaced Code"), w223, w227) -> (resulting string=w226:string)  [unwired: 2 in, 1 out]
        n93 = call "String Array Concatenate To String.vi"("insert last delimiter?"=FALSE, "Delimiter char"="\r\n", "Array String In"=w233) -> ("String"=w240:string)  [unwired: 8 in]
        n94 = call "String Indent Code.vi"("complete code"=w240, "actual nested level"=1) -> ("indented code"=w238:string)  [unwired: 9 in]
        n95 = Format Into String(format string="if (feedbackNodeInitBool_%d){\n%s\n}", w236, w238) -> (resulting string=w231:string)  [unwired: 2 in, 1 out]
        n96 = Concatenate Strings(w231, "\r\n", w230) -> (w232:string)
      }
      frame "Bundler" {
        w272 = refnum<vi> refnum  # Bundler
        # "Maybe forgot assign into output cluster."
        # "Transcripting Bundler, no all inputs has to be wired. We need to generate C++ structure items value assignement.\nwireUID_xxx = {.itemX = ???, .itemY = ???, ...};"
        n97 = To More Specific Class(target class=w272, reference=w271, error in=w270) -> (specific class reference=w269:refnum<vi>, error out=w268:errorcluster)
        n98 = case shown="Default" w265 {
          tunnel: w269 -> [w294 w323]
          tunnel: w268 -> [w293 w322]
          tunnel: [w275 w314] -> w267
          tunnel: [w279 w313] -> w266
          frame "Concatenate Strings" {
            # "Concatenate string function is class Bundler, so that's reason why its handler code is here."
            n99 = property class="Bundler"(reference=w294, error in=w293) -> (error out=w278:errorcluster, "InputTerms[]"=w292:refnum<vi>[], "Terms[]"=w283:refnum<vi>[])  [unwired: 1 out]
            n100 = for {
              tunnel: w292 -> [w303] mode=indexing
              tunnel: [w302] -> w291 mode=indexing
              tunnel: w278 -> [w301]
              tunnel: [w300] -> w277
              n101 = property class="Term"(reference=w303, error in=w301) -> (error out=w300:errorcluster, "Wire"=w302:refnum<vi>)  [unwired: 1 out]
            }
            n102 = for {
              tunnel: w283 -> [w299] mode=indexing
              tunnel: [w298] -> w286 mode=indexing if=w297
              tunnel: w278 -> [w296]
              tunnel: [w295] -> w274
              n103 = property class="Term"(reference=w299, error in=w296) -> (reference out=w298:refnum<vi>, error out=w295:errorcluster, "IsSource"=w297:bool)
            }
            n104 = call "Get Wires Info.vi"("connected\nwires refs."=w291) -> ("wires info cluster"=w290:T3)  [unwired: 10 in]
            n105 = Unbundle By Name(w290) -> ("wire labels"=w289:string[])
            n106 = Index Array(array=w286) -> (element=w285:refnum<vi>)  [unwired: 1 in]
            n107 = property class="Term"(reference=w285, error in=w274) -> (error out=w273:errorcluster, "Wire"=w284:refnum<vi>)  [unwired: 1 out]
            n108 = Merge Errors(w273, w277) -> (w276:errorcluster)
            n109 = call "Get Wire Info.vi"("Wire"=w284) -> ("wire label"=w281:string)  [unwired: 9 in, 1 out]
            n110 = call "String Array Concatenate To String.vi"("insert last delimiter?"=FALSE, "Delimiter char"=" + ", "Array String In"=w289) -> ("String"=w280:string)  [unwired: 8 in]
            n111 = Format Into String(format string="%s = %s;", error in=w276, w281, w280) -> (resulting string=w279:string, error out=w275:errorcluster)  [unwired: 1 in]
          }
          frame Default {
            # "Unbundler needs to look inside typedef cluster to know what types are items. Without this it will produce just one line, because it will retruns just datatype of top most cluster."
            # "Get wire output name."
            # "Handling normal Bundler."
            n112 = property class="Bundler"(reference=w323, error in=w322) -> (reference out=w321:refnum<vi>, error out=w320:errorcluster, "InputTerms[]"=w318:refnum<vi>[], "Terms[]"=w312:refnum<vi>[])
            n113 = for {
              tunnel: w312 -> [w326] mode=indexing
              tunnel: [w325] -> w311 mode=indexing if=w324
              n114 = property class="Term"(reference=w326) -> (reference out=w325:refnum<vi>, "IsSource"=w324:bool)  [unwired: 1 in, 1 out]
            }
            n115 = call "Cluster Bundler Get Typedef Terminal.vi"("error in (no error)"=w320, "GObject in"=w321) -> ("Terminal out"=w308:refnum<vi>)  [unwired: 8 in, 1 out]
            n116 = call "Cluster Make Typedef Elements Info.vi"("skip first typedef?"=TRUE, "Terminal in"=w308) -> ("Cluster elements names"=w307:string[])  [unwired: 5 in, 4 out]
            n117 = Index Array(array=w311) -> (element=w310:refnum<vi>)  [unwired: 1 in]
            n118 = property class="Term"(reference=w310) -> ("Wire"=w309:refnum<vi>)  [unwired: 1 in, 2 out]
            n119 = call "Get Wire Info.vi"("Wire"=w309) -> ("wire label"=w306:string)  [unwired: 9 in, 1 out]
            n120 = for {
              tunnel: w318 -> [w338] mode=indexing
              tunnel: w307 -> [w330] mode=indexing
              tunnel: [w328] -> w317 mode=indexing if=w333
              tunnel: w306 -> [w327]
              # "is wirec connected?"
              n121 = property class="Term"(reference=w338) -> (error out=w335:errorcluster, "Wire.UID"=w337:i32, "Wire"=w332:refnum<vi>)  [unwired: 1 in, 1 out]
              n122 = Greater Or Equal To 0?(x=w337) -> (x >= 0?=w336:bool)
              n123 = Not(x=w335) -> (.not. x?=w334:bool)
              n124 = call "Get Wire Info.vi"("Wire"=w332) -> ("wire label"=w329:string)  [unwired: 9 in, 1 out]
              n125 = And(x=w334, y=w336) -> (x .and. y?=w333:bool)
              n126 = Format Into String(format string="%s.%s = %s;", w327, w330, w329) -> (resulting string=w328:string)  [unwired: 2 in, 1 out]
            }
            n127 = call "String Array Concatenate To String.vi"("insert last delimiter?"=FALSE, "Delimiter char"="\r\n", "Array String In"=w317) -> ("String"=w315:string)  [unwired: 8 in]
            n128 = Format Into String(format string="%s //bundler", w315) -> (resulting string=w313:string, error out=w314:errorcluster)  [unwired: 2 in]
          }
        }
      }
      frame "Unbundler" {
        w360 = refnum<vi> refnum  # Unbundler
        # "Unbundler needs to look inside typedef cluster to know what types are items. Without this it will produce just one line, because it will retruns just datatype of top most cluster."
        # "output terminals of bundler are there even when not wired, so there would be same count of datatypes and output terminals"
        # "Maybe forgot assign into output cluster."
        # "Get INPUT terminal connected wire name. It's only one input terminal on Unbundler."
        # "Translating Unbundler, in C/C++ unbundler represents getting value from structure. Structure is in C/C++ sequentially stored in memory. We need to use general access to items as we don't have information about cluster (structure) items names, this information could be lost as wire is going out of case structure or any else structure, LabVIEW just store items datatypes, it's visible in context help when passing mouse through wires."
        n129 = To More Specific Class(target class=w360, reference=w357, error in=w356) -> (specific class reference=w359:refnum<vi>, error out=w358:errorcluster)
        n130 = property class="Unbundler"(reference=w359, error in=w358) -> (error out=w344:errorcluster, "Terms[]"=w353:refnum<vi>[], "OutputTerms[]"=w351:refnum<vi>[])  [unwired: 1 out]
        n131 = for {
          tunnel: w353 -> [w383] mode=indexing
          tunnel: [w382] -> w355 mode=indexing if=w380
          n132 = property class="Term"(reference=w383) -> (reference out=w382:refnum<vi>, "IsSource"=w381:bool)  [unwired: 1 in, 1 out]
          n133 = Not(x=w381) -> (.not. x?=w380:bool)
        }
        n134 = Index Array(array=w355) -> (element=w350:refnum<vi>)  [unwired: 1 in]
        n135 = property class="Term"(reference=w350) -> ("Wire"=w354:refnum<vi>)  [unwired: 1 in, 2 out]
        n136 = call "Cluster Make Typedef Elements Info.vi"("skip first typedef?"=TRUE, "Terminal in"=w350) -> ("Cluster elements datatypes"=w346:string[])  [unwired: 5 in, 4 out]
        n137 = call "Get Wire Info.vi"("Wire"=w354) -> ("wire label"=w352:string)  [unwired: 9 in, 1 out]
        n138 = for {
          tunnel: w352 -> [w373]
          tunnel: w351 -> [w378] mode=indexing
          tunnel: [w377] -> w349 mode=indexing if=w367
          tunnel: w346 -> [w370] mode=indexing
          shift-right: [w376] -> _
          shift-left: "" ("format string") -> [w363]
          # "counting index where to jump"
          # "Assign values to output wires connected to Unbundler.\nUnbundler has all items visible in LabVIEW block editor, so acess item is done using pointer (counting memory size using size() and acess memory space directly)"
          n139 = call "LabVIEW Datatype Prefix.vi"() -> ("datatype prefix"=w361:string)
          n140 = Concatenate Strings(w361, w370) -> (w362:string)
          n141 = property class="Term"(reference=w378) -> ("Wire"=w369:refnum<vi>)  [unwired: 1 in, 2 out]
          n142 = Format Into String(format string="*(%s*)", w362) -> (resulting string=w365:string)  [unwired: 2 in, 1 out]
          n143 = Format Into String(format string="+ sizeof(%s)", w362) -> (resulting string=w374:string)  [unwired: 2 in, 1 out]
          n144 = Format Into String(format string="((void*) &%s)", w373) -> (resulting string=w364:string)  [unwired: 2 in, 1 out]
          n145 = call "Get Wire Info.vi"("Wire"=w369) -> ("wire label"=w366:string)  [unwired: 9 in, 1 out]
          n146 = Empty String/Path?(string/path=w366) -> (empty?=w368:bool)
          n147 = Not(x=w368) -> (.not. x?=w367:bool)
          n148 = Concatenate Strings(w363, w374) -> (w376:string)
          n149 = Format Into String(format string="%s = (%s (%s %s));", w366, w365, w364, w363) -> (resulting string=w377:string)  [unwired: 2 in, 1 out]
        }
        n150 = call "String Array Concatenate To String.vi"("insert last delimiter?"=FALSE, "Delimiter char"="\r\n", "Array String In"=w349) -> ("String"=w342:string)  [unwired: 8 in]
        n151 = Format Into String(format string="/***** BEGIN  Unbundler *****/\n%s\n/***** END Unbundler *****/", w342) -> (resulting string=w341:string)  [unwired: 2 in, 1 out]
      }
      frame "NamedBundler" {
        w388 = refnum<vi> refnum  # NamedBundler
        # "Implementing this, there is problem, that I cannot relay on items name from LabVIEW so instead I have to use items position within structure, expecting that data are aligned without any space."
        n152 = To More Specific Class(target class=w388, reference=w391, error in=w390) -> (specific class reference=w387:refnum<vi>, error out=w389:errorcluster)
        n153 = disable-structure shown="Disabled" {
          disable-tunnel: w389 -> [w412 w442]
          disable-tunnel: w387 -> [w411 w448]
          disable-tunnel: [w402 w432] -> w386
          disable-tunnel: [w392 w423] -> w385
          frame Disabled {
            n154 = property class="NmdBndl" props=["ElemNms[]", "Terms[]", "InputTerms[]", "AvailElems[]"](reference=w411, error in=w412) -> (error out=w403:errorcluster, "ElemNms[]"=w399:string[], "Terms[]"=w407:refnum<vi>[], "InputTerms[]"=w401:refnum<vi>[])  [unwired: 2 out]
            n155 = for {
              tunnel: w401 -> [w419] mode=indexing
              tunnel: [w418] -> w400 mode=indexing
              n156 = property class="Term"(reference=w419) -> ("Wire"=w418:refnum<vi>)  [unwired: 1 in, 2 out]
            }
            n157 = for {
              tunnel: w407 -> [w422] mode=indexing
              tunnel: [w421] -> w406 mode=indexing if=w420
              n158 = property class="Term"(reference=w422) -> (reference out=w421:refnum<vi>, "IsSource"=w420:bool)  [unwired: 1 in, 1 out]
            }
            n159 = call "Get Wires Info.vi"("connected\nwires refs."=w400) -> ("wires info cluster"=w398:T3)  [unwired: 10 in]
            n160 = Index Array(array=w406) -> (element=w405:refnum<vi>)  [unwired: 1 in]
            n161 = Unbundle By Name(w398) -> ("wire labels"=w397:string[])
            n162 = for {
              tunnel: w399 -> [w414] mode=indexing
              tunnel: w397 -> [w416] mode=indexing
              tunnel: [w415] -> w396 mode=indexing
              n163 = call "String Correct Whitespaces.vi"("String in"=w414) -> ("String out"=w413:string)  [unwired: 10 in]
              n164 = Format Into String(format string=".%s = %s" ("Delimiter char"), w413, w416) -> (resulting string=w415:string)  [unwired: 2 in, 1 out]
            }
            n165 = property class="Term"(reference=w405) -> ("Wire"=w404:refnum<vi>)  [unwired: 1 in, 2 out]
            n166 = call "String Array Concatenate To String.vi"("insert last delimiter?"=FALSE, "Delimiter char"=",", "Array String In"=w396) -> ("String"=w394:string)  [unwired: 8 in]
            n167 = call "Get Wire Info.vi"("Wire"=w404) -> ("wire datatype"=w393:string, "wire label"=w395:string)  [unwired: 9 in]
            n168 = Format Into String(format string="%s = *(%s*) (new %s{%s}); //Bundler gen." ("Delimiter char"), error in=w403, w395, w393, w394) -> (resulting string=w392:string, error out=w402:errorcluster)  [unwired: 2 in]
          }
          frame Enabled {
            # "Assign input wire value into output wire."
            # "Getting output wire info."
            # "Input structure name."
            n169 = property class="NmdBndl"(reference=w448, error in=w442) -> (error out=w441:errorcluster, "AvailElems[]"=w445:string[], "ElemNms[]"=w446:string[], "InputTerms[]"=w447:refnum<vi>[], "Terms[]"=w455:refnum<vi>[])  [unwired: 1 out]
            n170 = for {
              tunnel: w455 -> [w492] mode=indexing
              tunnel: [w491] -> w453 mode=indexing if=w488
              tunnel: [w487] -> w450 mode=indexing if=w488
              tunnel: w441 -> [w490]
              tunnel: [w489] -> w440
              tunnel: [w487] -> w430 mode=indexing if=w486
              n171 = property class="Term"(reference=w492, error in=w490) -> (error out=w489:errorcluster, "Wire"=w487:refnum<vi>, "IsSource"=w488:bool, "Data Type"=w491:variant)  [unwired: 1 out]
              n172 = Not(x=w488) -> (.not. x?=w486:bool)
            }
            n173 = for {
              tunnel: w447 -> [w471] mode=indexing
              tunnel: [w470] -> w443 mode=indexing
              tunnel: w446 -> [w468] mode=indexing
              tunnel: w445 -> [w469]
              tunnel: [w467] -> w444 mode=indexing
              # "Getting index of\nitems inside cluster."
              # "Get values foritems which should be replaced."
              n174 = property class="Term"(reference=w471) -> ("Wire"=w470:refnum<vi>)  [unwired: 1 in, 2 out]
              n175 = Search 1D Array(1D array=w469, element=w468) -> (index of element=w467:i32)  [unwired: 1 in]
            }
            n176 = Index Array(array=w453) -> (element=w452:variant)  [unwired: 1 in]
            n177 = Index Array(array=w450) -> (element=w449:refnum<vi>)  [unwired: 1 in]
            n178 = Index Array(array=w430) -> (element=w431:refnum<vi>)  [unwired: 1 in]
            n179 = call "Get Wires Info.vi"("connected\nwires refs."=w443) -> ("wires info cluster"=w454:T3)  [unwired: 10 in]
            n180 = call "Get Wire Info.vi"("Wire"=w431) -> ("wire datatype"=w427:string, "wire label"=w428:string)  [unwired: 9 in]
            n181 = Unbundle By Name(w454) -> ("wire labels"=w438:string[], "wire terminals datatypes"=w437:string[][])
            n182 = call "Get Wire Info.vi"("Wire"=w449) -> ("wire label"=w429:string)  [unwired: 9 in, 1 out]
            n183 = call "Cluster Get Datatype From Variant.vi"("cluster variant in"=w452) -> ("cluster elements datatypes"=w451:string[])  [unwired: 9 in, 1 out]
            n184 = for {
              tunnel: w444 -> [w477] mode=indexing
              tunnel: w451 -> [w481]
              tunnel: w440 -> [w473]
              tunnel: [w473] -> w433
              tunnel: [w472] -> w439 mode=indexing
              # "Computes items memory index, counting it by items datatypes.\nCreates \"sizeof(int) + sizeof(String)\" ..."
              n185 = for {
                N: w477 -> [_]
                tunnel: w481 -> [w484] mode=indexing
                tunnel: [w483] -> w480 mode=indexing
                n186 = call "LabVIEW Datatype Prefix.vi"() -> ("datatype prefix"=w482:string)
                n187 = Format Into String(format string="sizeof(%s%s)", w482, w484) -> (resulting string=w483:string)  [unwired: 2 in, 1 out]
              }
              n188 = call "String Array Concatenate To String.vi"("insert last delimiter?"=FALSE, "Delimiter char"=" + ", "Array String In"=w480) -> ("String"=w475:string)  [unwired: 8 in]
              n189 = Equal To 0?(x=w477) -> (x = 0?=w476:bool)
              n190 = Select(t="0" ("Delimiter char"), s=w476, f=w475) -> (s? t:f=w472:string)
            }
            n191 = for {
              tunnel: [w465] -> w434 mode=indexing
              tunnel: w439 -> [w458] mode=indexing
              tunnel: w438 -> [w457] mode=indexing
              tunnel: w437 -> [w463] mode=indexing
              tunnel: w429 -> [w460]
              tunnel: [w464] -> w432
              tunnel: w433 -> [w456]
              # "Replacing values of selected items, using pointer arithmetic to access items.\nThere is mistake in LabVIEW (probably it als doesn't use names but computes memory location manually based on items datatypes)."
              n192 = call "LabVIEW Datatype Prefix.vi"() -> ("datatype prefix"=w462:string)
              n193 = Index Array(array=w463) -> (element=w461:string)  [unwired: 1 in]
              n194 = Concatenate Strings(w462, w461) -> (w459:string)
              n195 = Format Into String(format string="*((%s*) &%s + %s) =  %s;" ("Delimiter char"), error in=w456, w459, w460, w458, w457) -> (resulting string=w465:string, error out=w464:errorcluster)  [unwired: 1 in]
            }
            n196 = Format Into String(format string="%s = *(%s*) &%s;\\n" ("Delimiter char"), w428, w427, w429) -> (resulting string=w425:string)  [unwired: 2 in, 1 out]
            n197 = call "String Array Concatenate To String.vi"("insert last delimiter?"=TRUE, "Delimiter char"="\r\n", "Array String In"=w434) -> ("String"=w424:string)  [unwired: 8 in]
            n198 = Concatenate Strings(w425, w424) -> (w423:string)
          }
        }
      }
      frame "NamedUnbundler" {
        w517 = refnum<vi> refnum  # NamedUnbundler
        # "Input structure name."
        # "Generate code to get item from structure, but because we cannot be sure cluster item names we have to use item access through pointer because datatypes of cluster are known.\nResult code is:\nitem1 = *(LV_Cluster_int_String*) ((void*) &inputStruct + 0);\nitem2 = *(LV_Cluster_int_String*) ((void*) &inputStruct + sizeof(int));"
        n199 = To More Specific Class(target class=w517, reference=w520, error in=w519) -> (specific class reference=w516:refnum<vi>, error out=w518:errorcluster)
        n200 = property class="NmdUnbndl"(reference=w516, error in=w518) -> (error out=w515:errorcluster, "AvailElems[]"=w501:string[], "ElemNms[]"=w502:string[], "OutputTerms[]"=w512:refnum<vi>[], "Terms[]"=w513:refnum<vi>[])  [unwired: 1 out]
        n201 = for {
          tunnel: w513 -> [w554] mode=indexing
          tunnel: [w552] -> w505 mode=indexing if=w550
          tunnel: [w551] -> w496 mode=indexing if=w550
          n202 = property class="Term"(reference=w554) -> ("Wire"=w551:refnum<vi>, "IsSource"=w553:bool, "Data Type"=w552:variant)  [unwired: 1 in, 2 out]
          n203 = Not(x=w553) -> (.not. x?=w550:bool)
        }
        n204 = for {
          tunnel: w512 -> [w549] mode=indexing
          tunnel: [w548] -> w511 mode=indexing
          tunnel: w502 -> [w546] mode=indexing
          tunnel: w501 -> [w547]
          tunnel: [w545] -> w500 mode=indexing
          # "Getting index of\nitems inside cluster."
          # "Traversing just output wired items and remember their indexes to be able get their names from Available Elements[]"
          n205 = property class="Term"(reference=w549) -> ("Wire"=w548:refnum<vi>)  [unwired: 1 in, 2 out]
          n206 = Search 1D Array(1D array=w547, element=w546) -> (index of element=w545:i32)  [unwired: 1 in]
        }
        n207 = call "Get Wires Info.vi"("connected\nwires refs."=w511) -> ("wires info cluster"=w510:T3)  [unwired: 10 in]
        n208 = Index Array(array=w505) -> (element=w504:variant)  [unwired: 1 in]
        n209 = Index Array(array=w496) -> (element=w495:refnum<vi>)  [unwired: 1 in]
        n210 = Unbundle By Name(w510) -> ("wire labels"=w509:string[], "wire terminals datatypes"=w497:string[][])
        n211 = call "Get Wire Info.vi"("Wire"=w495) -> ("wire label"=w494:string)  [unwired: 9 in, 1 out]
        n212 = call "Cluster Get Datatype From Variant.vi"("cluster variant in"=w504) -> ("cluster elements datatypes"=w499:string[])  [unwired: 9 in, 1 out]
        n213 = for {
          tunnel: w500 -> [w525] mode=indexing
          tunnel: w499 -> [w529]
          tunnel: [w522] -> w498 mode=indexing
          # "Computes items memory index, counting it by items datatypes."
          n214 = for {
            N: w525 -> [_]
            tunnel: w529 -> [w532] mode=indexing
            tunnel: [w531] -> w528 mode=indexing
            n215 = call "LabVIEW Datatype Prefix.vi"() -> ("datatype prefix"=w530:string)
            n216 = Format Into String(format string="sizeof(%s%s)", w530, w532) -> (resulting string=w531:string)  [unwired: 2 in, 1 out]
          }
          n217 = call "String Array Concatenate To String.vi"("insert last delimiter?"=FALSE, "Delimiter char"=" + ", "Array String In"=w528) -> ("String"=w523:string)  [unwired: 8 in]
          n218 = Equal To 0?(x=w525) -> (x = 0?=w524:bool)
          n219 = Select(t="0" ("Delimiter char"), s=w524, f=w523) -> (s? t:f=w522:string)
        }
        n220 = for {
          shift-right: [w542] -> w514
          shift-left: w515 -> [w538]
          tunnel: [w543] -> w503 mode=indexing
          tunnel: w498 -> [w539] mode=indexing
          tunnel: w509 -> [w541] mode=indexing
          tunnel: w497 -> [w540] mode=indexing
          tunnel: w494 -> [w537]
          # "Generating item value access using pointer arithmetics, we know cluster item datatypes so we have to just add size of each item from beginning of cluster and then retype this value to correct datatype :)"
          n221 = call "LabVIEW Datatype Prefix.vi"() -> ("datatype prefix"=w536:string)
          n222 = Index Array(array=w540) -> (element=w535:string)  [unwired: 1 in]
          n223 = Concatenate Strings(w536, w535) -> (w534:string)
          n224 = Format Into String(format string="%s = *(%s*) ((void*) &%s + %s);" ("Delimiter char"), error in=w538, w541, w534, w537, w539) -> (resulting string=w543:string, error out=w542:errorcluster)  [unwired: 1 in]
        }
        n225 = call "String Array Concatenate To String.vi"("insert last delimiter?"=TRUE, "Delimiter char"="\r\n", "Array String In"=w503) -> ("String"=w506:string)  [unwired: 8 in]
      }
      frame "FlatSequenceFrame" {
        w574 = refnum<vi> refnum  # FlatSequenceFrame
        # "No indentation, frames are like normal part of code. This is here just to show that idea :)"
        # "Under this node name see transcriptor each frame of FlatSequence. There is object FlatSequence, which is daughter object of GObject and sibling of Node, but property FiringOrder returns array of Nodes, even FlatSequenceFrame is not daughter of GObject but Generic, I don't know how it's possible that this ibject pass between all others Node inside array, but this is how to handle it.\nValues assignements for inside wires is done in steps 1. and 2. there are definition how to handle tunnels for FlatSequenceFrame."
        n226 = To More Specific Class(target class=w574, reference=w575, error in=w571) -> (specific class reference=w573:refnum<vi>, error out=w570:errorcluster)
        n227 = property on="Property Node" class="FlatSeqFrame"(reference=w573, error in=w570) -> (error out=w566:errorcluster, "Diagram"=w572:refnum<vi>, "OuterTunnels[]"=w560:refnum<vi>[])  [unwired: 1 out]
        n228 = for {
          tunnel: w560 -> [w592] mode=indexing
          tunnel: [w584] -> w559 mode=indexing if=w577
          w579 = 0 ("index (row)")
          # "don't generate assignements for error wire"
          # "Generating output values assignements for output tunnels from frame. If outside tunnel is on right side of sequence is recognized by isSource? property."
          n229 = property on="Property Node" class="FlatSeqOutTun"(reference=w592) -> ("OuterTerminal.Wire"=w591:refnum<vi>, "InnerTerminal.Wire"=w590:refnum<vi>, "OuterTerminal.IsSource"=w583:bool)  [unwired: 1 in, 2 out]
          n230 = Build Array(w591, w590) -> (w589:refnum<vi>[])
          n231 = call "Get Wires Info.vi"("connected\nwires refs."=w589) -> ("wires info cluster"=w588:T3)  [unwired: 10 in]
          n232 = Unbundle By Name(w588) -> ("wire labels"=w582:string[], "wire terminals datatypes"=w581:string[][])
          n233 = Index Array(array=w582) -> (element #1=w586:string, element #2=w585:string)  [unwired: 2 in]
          n234 = Index Array(array=w581, index (row)=w579, index (col)=w579) -> (element=w578:string)
          n235 = Not Equal?(x=w578, y="error") -> (x != y?=w576:bool)
          n236 = Format Into String(format string="%s = %s;", w586, w585) -> (resulting string=w584:string)  [unwired: 2 in, 1 out]
          n237 = And(x=w576, y=w583) -> (x .and. y?=w577:bool)
        }
        n238 = call "Transcriptor LabVIEW to C code Engine 2.vi"("Error In"=w566, "List Reentrant VIs"=w555, "Diagram in"=w572) -> ("error out"=w565:errorcluster, "output cluster"=w564:T1, "transcripted code"=w569:string)  [unwired: 4 in, 2 out]
        n239 = call "String Indent Code.vi"("complete code"=w569, "actual nested level"=0) -> ("indented code"=w562:string)  [unwired: 9 in]
        n240 = Build Array(w564) -> (w563:T1[])
        n241 = call "String Array Concatenate To String.vi"("insert last delimiter?"=FALSE, "Delimiter char"="\r\n", "Array String In"=w559) -> ("String"=w556:string)  [unwired: 8 in]
        n242 = Format Into String(format string="/* FlatSequenceFrame */\n%s\n%s //frame output assignemnts\n/* end FlatSequenceFrame */", w562, w556) -> (resulting string=w561:string)  [unwired: 2 in, 1 out]
      }
      frame "StaticVIReference" {
        w613 = refnum<vi> refnum  # SubVI
        w621 = refnum<vi> refnum  # StaticVIReference
        # "CHECK HOW IS THIS IMPLEMENTED,\nthis is nonesens, need to revalide what I wanted to do"
        n243 = To More Specific Class(target class=w621, reference=w620, error in=w619) -> (specific class reference=w615:refnum<vi>, error out=w618:errorcluster)
        n244 = property class="StatVIRef"(reference=w615, error in=w618) -> (error out=w606:errorcluster, "Path"=w612:path, "UID"=w595:i32)  [unwired: 1 out]
        n245 = New VI Object(vi object class=w613, owner refnum=w614, position/next to=T2 {"Horizontal"=10, "Vertical"=0} ("location"), 6:w612, 8:w606) -> (object refnum=w609:refnum<vi>, 0:w610:errorcluster)  [unwired: 3 in]
        n246 = call "SubVI Translate.vi"("error in (no error)"=w610, "SubVI in"=w609) -> ("error out"=w611:errorcluster, "transcripted code"=w607:string, "transcriptor cluster"=w603:T1)  [unwired: 6 in, 1 out]
        n247 = Format Into String(format string="StaticVIReferenceUID_%d", w595) -> (resulting string=w594:string)  [unwired: 2 in, 1 out]
        n248 = invoke class="SubVI" method="Delete"(reference=w609, error in=w611) -> (error out=w605:errorcluster)  [unwired: 1 in, 2 out]
        n249 = Unbundle By Name(w603) -> ("Defines"=w600:string[], "Includes"=w602:string[])
        n250 = Format Into String(format string="/***** interruption *****/\nvoid %s(){\n%s\n}\n/***** end interruption *****/", w594, w607) -> (resulting string=w599:string)  [unwired: 2 in, 1 out]
        n251 = Build Array (concatenate)(w599, w600) -> (w601:string[])
        n252 = Bundle By Name(cluster=w603, "Defines"=w601, "Includes"=w602) -> (w604:T1)
        n253 = Build Array(w604) -> (w616:T1[])
        n254 = Format Into String(format string="/* StaticVIReference transcripted, ISR name \"%s\" */", w594) -> (resulting string=w597:string)  [unwired: 2 in, 1 out]
      }
      frame "SharedVariableNode" {
        w647 = refnum<vi> refnum  # SharedVariableNode
        # "Connected wirte to write input/read input."
        # "If there are multiple assignements into global var, but different datatypes it will generate definition for both, this error occurs at compilation time, what is basically right and user will see that there are more declarations for same global and can find it by datatype or something.\nAt least will have some info what to look for :)"
        # "Need to add prefix, auxiliary functions for transcriptor are returning datatype in raw form, so if it has to be transcripted it needs to start with prefix for datatypes (it's something like LVDatatype, I prepared VI for it)."
        # "Variables represent global variables, so they are placed at definitions place in the beginning of file."
        # "Doesn't matter if variable for write or read, input/output terminal has index 0 (I made for loop and let written terminals names into code, variable terminal was in both cases at index 0)."
        # "Using negative looking, look for \\ (slash) which is not followed by any other slash and after take all characters until end of string."
        # "SharedVariables are in transcriptor used to create global variables, because they are treat in LabVIEW in similar way like global variables in C/C++.\nIt's not possible to store class into variable, so I have to little go around this, because I want to be able store them because user defined datatypes (otherwise user will be constrained by this mechanism just to LabVIEW basic datatypes). For this I'm using variant datatype. User has to wire when writing into variable wire with class datatype (so that wire which is going into variable has to be other color than purple for variant) and there has to be coertion dot ont variable input terminal. \n\nGlobal variables declaration are created with datatype based on wires connected to variables other than variants. So if we want to have custom datatype global variable we have to reate variant global variable and then somewhere in code write into this variable specific class with required datatype and this global variable will be created."
        n255 = To More Specific Class(target class=w647, reference=w648, error in=w649) -> (specific class reference=w646:refnum<vi>, error out=w645:errorcluster)
        n256 = property class="SharedVariableNode"(reference=w646, error in=w645) -> (error out=w639:errorcluster, "Label.Text"=w632:string, "Terms[]"=w634:refnum<vi>[], "Write?"=w631:bool)  [unwired: 1 out]
        n257 = Index Array(array=w634, index=0) -> (element=w640:refnum<vi>)
        n258 = property class="Term"(reference=w640, error in=w639) -> (error out=w636:errorcluster, "Wire"=w629:refnum<vi>, "Data Type"=w628:variant)  [unwired: 1 out]
        n259 = xnode "Match Regular Expression"("input string"=w632, "regular expression"="(?!.*\\\\).*$") -> ("whole match"=w630:string)  [unwired: 4 in, 4 out]
        n260 = call "Get Wire Info.vi"("Wire"=w629) -> ("wire datatype"=w622:string, "wire label"=w623:string)  [unwired: 9 in]
        n261 = call "Get Variant Data Type.vi"("Variant in"=w628) -> ("Data Types[]"=w627:string[])  [unwired: 9 in, 1 out]
        n262 = call "String Array Concatenate To String.vi"("Array String In"=w627) -> ()  [unwired: 10 in, 1 out]
        n263 = Not Equal?(x="LV Variant", y=w622) -> (x != y?=w624:bool)
        n264 = case shown="True" w624 {
          tunnel: ["" w655] -> w637
          tunnel: w630 -> [_ w653]
          tunnel: w622 -> [_ w652]
          frame False {
            # "If global variable is read it's into variant wire, later it has to be retyped, but this definition for LV Varaint is not put into list."
          }
          frame True {
            # "Put global var declaration into list."
            n265 = call "LabVIEW Datatype Prefix.vi"() -> ("datatype prefix"=w654:string)
            n266 = Concatenate Strings(w654, w652) -> (w651:string)
            n267 = Format Into String(format string="%s %s;", w651, w653) -> (resulting string=w655:string)  [unwired: 2 in, 1 out]
          }
        }
        n268 = Build Array(w637) -> (w638:string[])
        n269 = case shown="False" w631 {
          tunnel: w623 -> [w657 w669]
          tunnel: w630 -> [w658 w661]
          tunnel: [w660 w668] -> w626
          tunnel: w624 -> [_ w666]
          frame True {
            # "Write into global var."
            n270 = Format Into String(format string="%s = %s;", w658, w657) -> (resulting string=w660:string)  [unwired: 2 in, 1 out]
          }
          frame False {
            # "Read from global var, if reading into Variant wire then retype it to Variant."
            n271 = call "LabVIEW Datatype Prefix.vi"() -> ("datatype prefix"=w663:string)
            n272 = Format Into String(format string="(%sLV Variant) &%s" ("string"), w663, w661) -> (resulting string=w662:string)  [unwired: 2 in, 1 out]
            n273 = Select(t=w661, s=w666, f=w662) -> (s? t:f=w665:string)
            n274 = Format Into String(format string="%s = %s;", w669, w665) -> (resulting string=w668:string)  [unwired: 2 in, 1 out]
          }
        }
        n275 = Bundle By Name(cluster=T1 {"Defines"=[], "Includes"=[], "C code"="", "temp"=[], "temp 2"=[], "wires with breakpoints"=[]} ("input cluster"), "Defines"=w638) -> (w641:T1)
        n276 = Build Array(w641) -> (w642:T1[])
      }
    }
  }
  "feedback assignments" <- w8
  "error out" <- w7
  "transcriptor cluster" <- w3
  "transcripted C code" <- w5
